vi "StandardStateMachine.vi"() -> ()   [LabVIEW 2020]
doc: "Use this template to build a standard state machine design pattern. Each state executes code and determines which state to transition to. Contrast this design pattern with the User Interface Event Handler pattern, in which code executes in response to user actions. Contrast this design pattern also with the Queued Message Handler pattern, in which each message handling code can queue zero or more new messages."
uses:
  StateMachineStates.ctl
panel:
  in  "stop":bool
  out "error out":errorcluster
  in  "error in":errorcluster
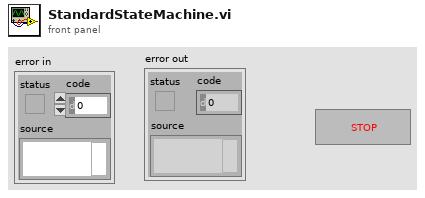
[diagram p1: front panel]
types:
  T1 = typedef "StateMachineStates.ctl" = enum16{"Initialize", "Idle", "Execute", "STOP"}
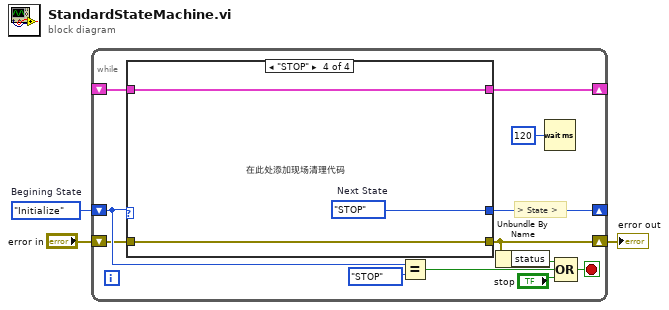
[diagram p0: block diagram]
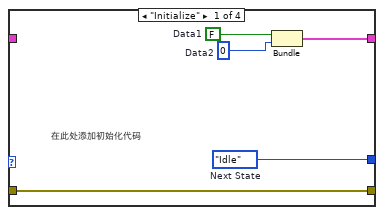
[diagram p2: hidden frame]
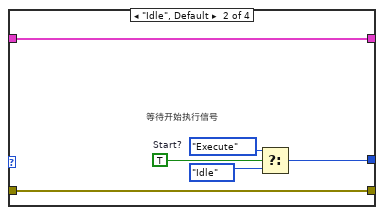
[diagram p3: hidden frame]
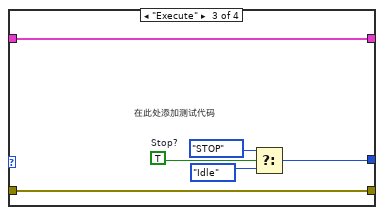
[diagram p4: hidden frame]
diagram:
  w3 = StateMachineStates."Initialize"  # Begining State
  n1 = while {
    shift-right: [w13] -> _
    shift-left: w3 -> [w14]
    shift-right: [w7] -> w1
    shift-left: "error in" -> [w8]
    shift-right: [w4] -> _
    shift-left: _ -> [w5]
    stop <- w10 stop-if-true
    # "> State >"
    n2 = case shown="\"STOP\"" w14 {
      tunnel: [w20 w23 w29 w35] -> w13
      tunnel: w8 -> [w19 w26 w30 w34]
      tunnel: [w19 w26 w30 w34] -> w7
      tunnel: w5 -> [_ w21 w27 w33]
      tunnel: [w17 w21 w27 w33] -> w4
      frame "Initialize" {
        w16 = 0  # Data2
        w18 = FALSE  # Data1
        w20 = StateMachineStates."Idle"  # Next State
        # "在此处添加初始化代码"
        n3 = Bundle("Data1"=w18, "Data2"=w16) -> (w17:cluster{"Data1":bool, "Data2":i32})  [unwired: 1 in]
      }
      frame "Idle", Default {
        w22 = TRUE  # Start?
        # "等待开始执行信号"
        n4 = Select(t=StateMachineStates."Execute" ("Next State"), s=w22, f=StateMachineStates."Idle" ("Next State")) -> (s? t:f=w23:T1)
      }
      frame "Execute" {
        w28 = TRUE  # Stop?
        # "在此处添加测试代码"
        n5 = Select(t=StateMachineStates."STOP" ("Next State"), s=w28, f=StateMachineStates."Idle" ("Next State")) -> (s? t:f=w29:T1)
      }
      frame "STOP" {
        w35 = StateMachineStates."STOP"  # Next State
        # "在此处添加现场清理代码"
      }
    }
    n6 = Equal?(x=w14, y=StateMachineStates."STOP" ("States")) -> (x = y?=w9:bool)
    n7 = Unbundle By Name(w7) -> ("status"=w6:bool)
    n8 = Wait (ms)(milliseconds to wait=u32 120) -> ()  [unwired: 1 out]
    n9 = Compound Arithmetic op=OR(w6, w9, "stop") -> (w10:bool)
  }
  "error out" <- w1
